vi "获取仪器状态.vi"(8 "error in (no error)":errorcluster caption="错误输入（无错误）", 11 "参数":enum16{"氨氮", "总磷", "总氮", "CODMn", "CODcr"}(ring)) -> (0 "error out":errorcluster caption="错误输出", 3 "仪器状态":enum16{"待机", "运行"}(ring))   [LabVIEW 2016, in "质控单元.lvlib"]
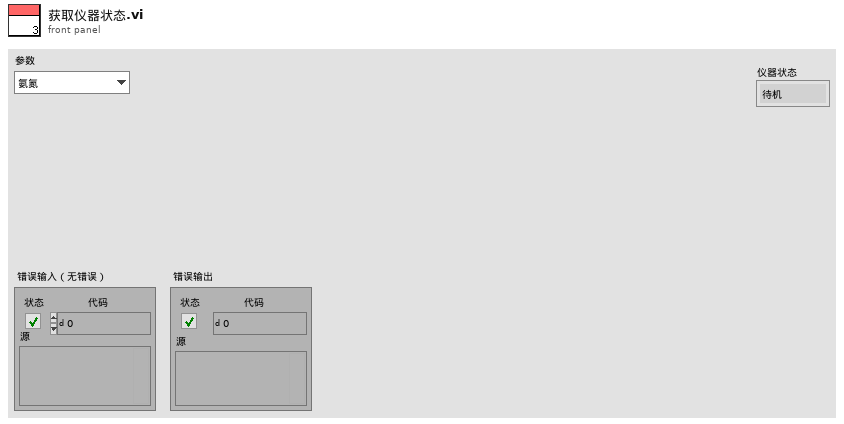
[diagram p1: front panel]
types:
  T1 = cluster{"系统时间":timestamp, "工作状态":enum16{"空闲", "水样测试", "标样核查", "零点核查", "跨度核查", "空白测试", "平行样测试", "加标回收", "空白校准", "标样校准", "初始化（清洗）"}, "测量模式":enum16{"待机", "连续模式", "周期模式", "定点模式", "受控模式", "手动模式"}, "告警代码":enum16{"无告警", "缺试剂告警", "缺水样告警", "缺蒸馏水告警", "缺标液告警", "仪表漏液告警", "标定异常告警", "超量程告警", "加热异常", "低试剂预警", "超上限告警", "超下限告警", "仪表内部其他异常", "滴定异常告警", "电极异常告警", "量程切换告警", "参数设置告警", "PH电极电位异常", "电导率电极异常", "浊度光度异常", "溶解氧电极异常", "溶解氧光强异常", "温度异常告警", "PH异常告警", "溶解氧异常告警", "电导率异常告警", "浊度异常告警", "叶绿素异常告警", "藻密度异常告警", "蓝绿藻异常告警", "ORP异常告警", "氨氮异常告警", "清洁刷异常告警", "SD卡异常告警", "蓝牙异常告警", "Wifi异常告警", "流程异常告警"}, "故障代码":enum16{"无故障", "电机故障", "温度故障", "通讯故障", "滴定故障"}, "日志代码":u16, "软件版本":u16, "F0":sgl, "F1":sgl, "F2":sgl, "F3":sgl, "T":sgl, "H":sgl, "id":u16, "flowid":u16, "量程":u16, "总磷控温温度1":sgl, "营养盐控温温度2":sgl, "ADC":sgl}
  T2 = enum16{"空闲", "水样测试", "标样核查", "零点核查", "跨度核查", "空白测试", "平行样测试", "加标回收", "空白校准", "标样校准", "初始化（清洗）"}
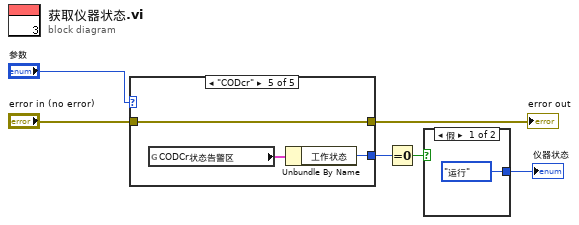
[diagram p0: block diagram]
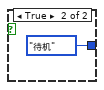
[diagram p2: hidden frame]
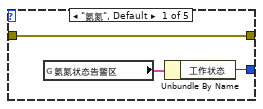
[diagram p3: hidden frame]
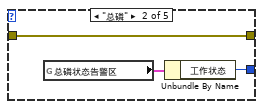
[diagram p4: hidden frame]
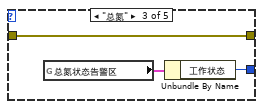
[diagram p5: hidden frame]
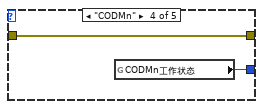
[diagram p6: hidden frame]
diagram:
  n1 = case shown="\"CODcr\"" "参数" {
    tunnel: [w8 w11 w14 w17 w19] -> w5
    tunnel: "error in (no error)" -> [w7 w10 w13 w16 w18]
    tunnel: [w7 w10 w13 w16 w18] -> w1
    frame "氨氮", Default {
      n2 = global read "与氨氮交互全局.vi" "氨氮状态告警区"() -> (w9:T1)
      n3 = Unbundle By Name(w9) -> ("工作状态"=w8:T2)
    }
    frame "总磷" {
      n4 = global read "与总磷交互全局.vi" "总磷状态告警区"() -> (w12:T1)
      n5 = Unbundle By Name(w12) -> ("工作状态"=w11:T2)
    }
    frame "总氮" {
      n6 = global read "与总氮交互全局.vi" "总氮状态告警区"() -> (w15:T1)
      n7 = Unbundle By Name(w15) -> ("工作状态"=w14:T2)
    }
    frame "CODMn" {
      n8 = global read "与CODMn交互全局.vi" "CODMn工作状态"() -> (w17:T2)
    }
    frame "CODcr" {
      n9 = global read "与CODCr交互全局.vi" "CODCr状态告警区"() -> (w20:T1)
      n10 = Unbundle By Name(w20) -> ("工作状态"=w19:T2)
    }
  }
  "error out" <- w1
  n11 = Equal To 0?(x=w5) -> (x = 0?=w4:bool)
  n12 = case shown="假" w4 {
    tunnel: [enum16{"待机", "运行"}."运行" ("仪器状态") enum16{"待机", "运行"}."待机" ("仪器状态")] -> w3
    frame False {
    }
    frame True {
    }
  }
  "仪器状态" <- w3
